vi "test-Coordinate-System-Test2.vi"() -> (3 "All tests passed":bool)   [LabVIEW 2019]
uses:
  <vilib>/Rock Robotics/WPI/ThirdParty/JAS_Junk/TrajLib/CoordAxis_N.vi
  <vilib>/Rock Robotics/WPI/ThirdParty/JAS_Junk/TrajLib/CoordSystem_New.vi
  <vilib>/Rock Robotics/WPI/ThirdParty/JAS_Junk/TrajLib/CoordAxis_E.vi
  <vilib>/Rock Robotics/WPI/ThirdParty/JAS_Junk/TrajLib/CoordAxis_D.vi
  <vilib>/Rock Robotics/WPI/ThirdParty/JAS_Junk/TrajLib/Conv_Deg_Radians.vi
  <vilib>/Rock Robotics/WPI/ThirdParty/JAS_Junk/TrajLib/Quaternion_New.vi
  <vilib>/Rock Robotics/WPI/ThirdParty/JAS_Junk/TrajLib/Translation3d_Create.vi
  <vilib>/Rock Robotics/WPI/ThirdParty/JAS_Junk/TrajLib/Pose3d_New_Trans3dRot3d.vi
  <vilib>/Rock Robotics/WPI/ThirdParty/JAS_Junk/TrajLib/Rotation3d_Minus.vi
  <vilib>/Rock Robotics/WPI/ThirdParty/JAS_Junk/TrajLib/Translation3d_Create_Default.vi
  <vilib>/Rock Robotics/WPI/ThirdParty/JAS_Junk/TrajLib/Pose3d_RelativeTo.vi
  <vilib>/Rock Robotics/WPI/ThirdParty/JAS_Junk/TrajLib/CoordAxis_New.vi
  <vilib>/Rock Robotics/WPI/ThirdParty/JAS_Junk/TrajLib/MatBuilder_Create.vi
  <vilib>/Rock Robotics/WPI/ThirdParty/JAS_Junk/TrajLib/Matrix_AssignBlock.vi
  <vilib>/Rock Robotics/WPI/ThirdParty/JAS_Junk/TrajLib/Matrix_Transpose.vi
  <vilib>/Rock Robotics/WPI/ThirdParty/JAS_Junk/TrajLib/Matrix_Ident.vi
  <vilib>/Rock Robotics/WPI/ThirdParty/JAS_Junk/TrajLib/Matrix_IsEqual.vi
  <vilib>/Analysis/baseanly.llb/A x B.vi
  <vilib>/Analysis/baseanly.llb/Real A x B.vi
  <vilib>/Rock Robotics/WPI/ThirdParty/JAS_Junk/TrajLib/Rotation3d_Create_Quaternion.vi
  <vilib>/Rock Robotics/WPI/ThirdParty/JAS_Junk/TrajLib/Rotation3d_UnaryMinus.vi
  <vilib>/Rock Robotics/WPI/ThirdParty/JAS_Junk/TrajLib/Rotation3d_RotateBy.vi
  <vilib>/Rock Robotics/WPI/ThirdParty/JAS_Junk/TrajLib/Transform3d_Create_Pose3dPose3d.vi
  <vilib>/Rock Robotics/WPI/ThirdParty/JAS_Junk/TrajLib/Transform3d_GetRotation3d.vi
  <vilib>/Rock Robotics/WPI/ThirdParty/JAS_Junk/TrajLib/Transform3d_GetTranslation3d.vi
  <vilib>/Rock Robotics/WPI/ThirdParty/JAS_Junk/TrajLib/Rotation3d_GetQuaterion.vi
  <vilib>/Rock Robotics/WPI/ThirdParty/JAS_Junk/TrajLib/Quaternion_Equals.vi
  <vilib>/Rock Robotics/WPI/ThirdParty/JAS_Junk/TrajLib/MatrixHelper_CoerceSize.vi
  <vilib>/Rock Robotics/WPI/ThirdParty/JAS_Junk/TrajLib/Quaternion_Normalize.vi
  <vilib>/Rock Robotics/WPI/ThirdParty/JAS_Junk/TrajLib/Quaternion_Inverse.vi
  <vilib>/Rock Robotics/WPI/ThirdParty/JAS_Junk/TrajLib/Quaternion_Times.vi
  <vilib>/Rock Robotics/WPI/ThirdParty/JAS_Junk/TrajLib/Transform3d_Create_Trans3dRot3d.vi
  <vilib>/Rock Robotics/WPI/ThirdParty/JAS_Junk/TrajLib/Translation3d_Minus.vi
  <vilib>/Rock Robotics/WPI/ThirdParty/JAS_Junk/TrajLib/Translation3d_RotateBy.vi
  <vilib>/Rock Robotics/WPI/ThirdParty/JAS_Junk/TrajLib/Quaternion_New_Default.vi
  <vilib>/Rock Robotics/WPI/ThirdParty/JAS_Junk/TrajLib/Quaternion_Get_All.vi
  <vilib>/Analysis/7linalg.llb/Create Special Matrix.vi
  <vilib>/Analysis/7linalg.llb/Create Special Real Matrix.vi
  <vilib>/Analysis/Matrix/Numeric/Conversions/Array To Matrix.vi
  <vilib>/Analysis/Matrix/Numeric/Conversions/Array To Matrix - RA.vi
  <vilib>/Rock Robotics/WPI/ThirdParty/JAS_Junk/TrajLib/Trajectory_Library.lvlib
panel:
  out "Test 4":bool
  out "Test 3":bool
  out "Test 2":bool
  out "Test 1":bool
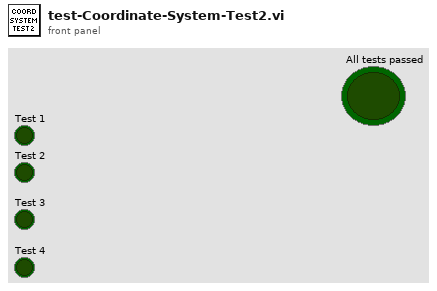
[diagram p1: front panel]
types:
  T1 = typedef "Trajectory_Library.lvlib/ROTATION3D.ctl" = cluster{"Q_quaternion":T2}
  T2 = typedef "Trajectory_Library.lvlib/QUATERNION.ctl" = cluster{"R":dbl, "V":dbl[]}
  T3 = typedef "Trajectory_Library.lvlib/POSE3D.ctl" = cluster{"Translation3d":T4, "Rotation3d":T1}
  T4 = typedef "Trajectory_Library.lvlib/TRANSLATION3D.ctl" = cluster{"X":dbl, "Y":dbl, "Z":dbl}
  T5 = typedef "Trajectory_Library.lvlib/COORDINATE_SYSTEM.ctl" = cluster{"Rotation":T1}
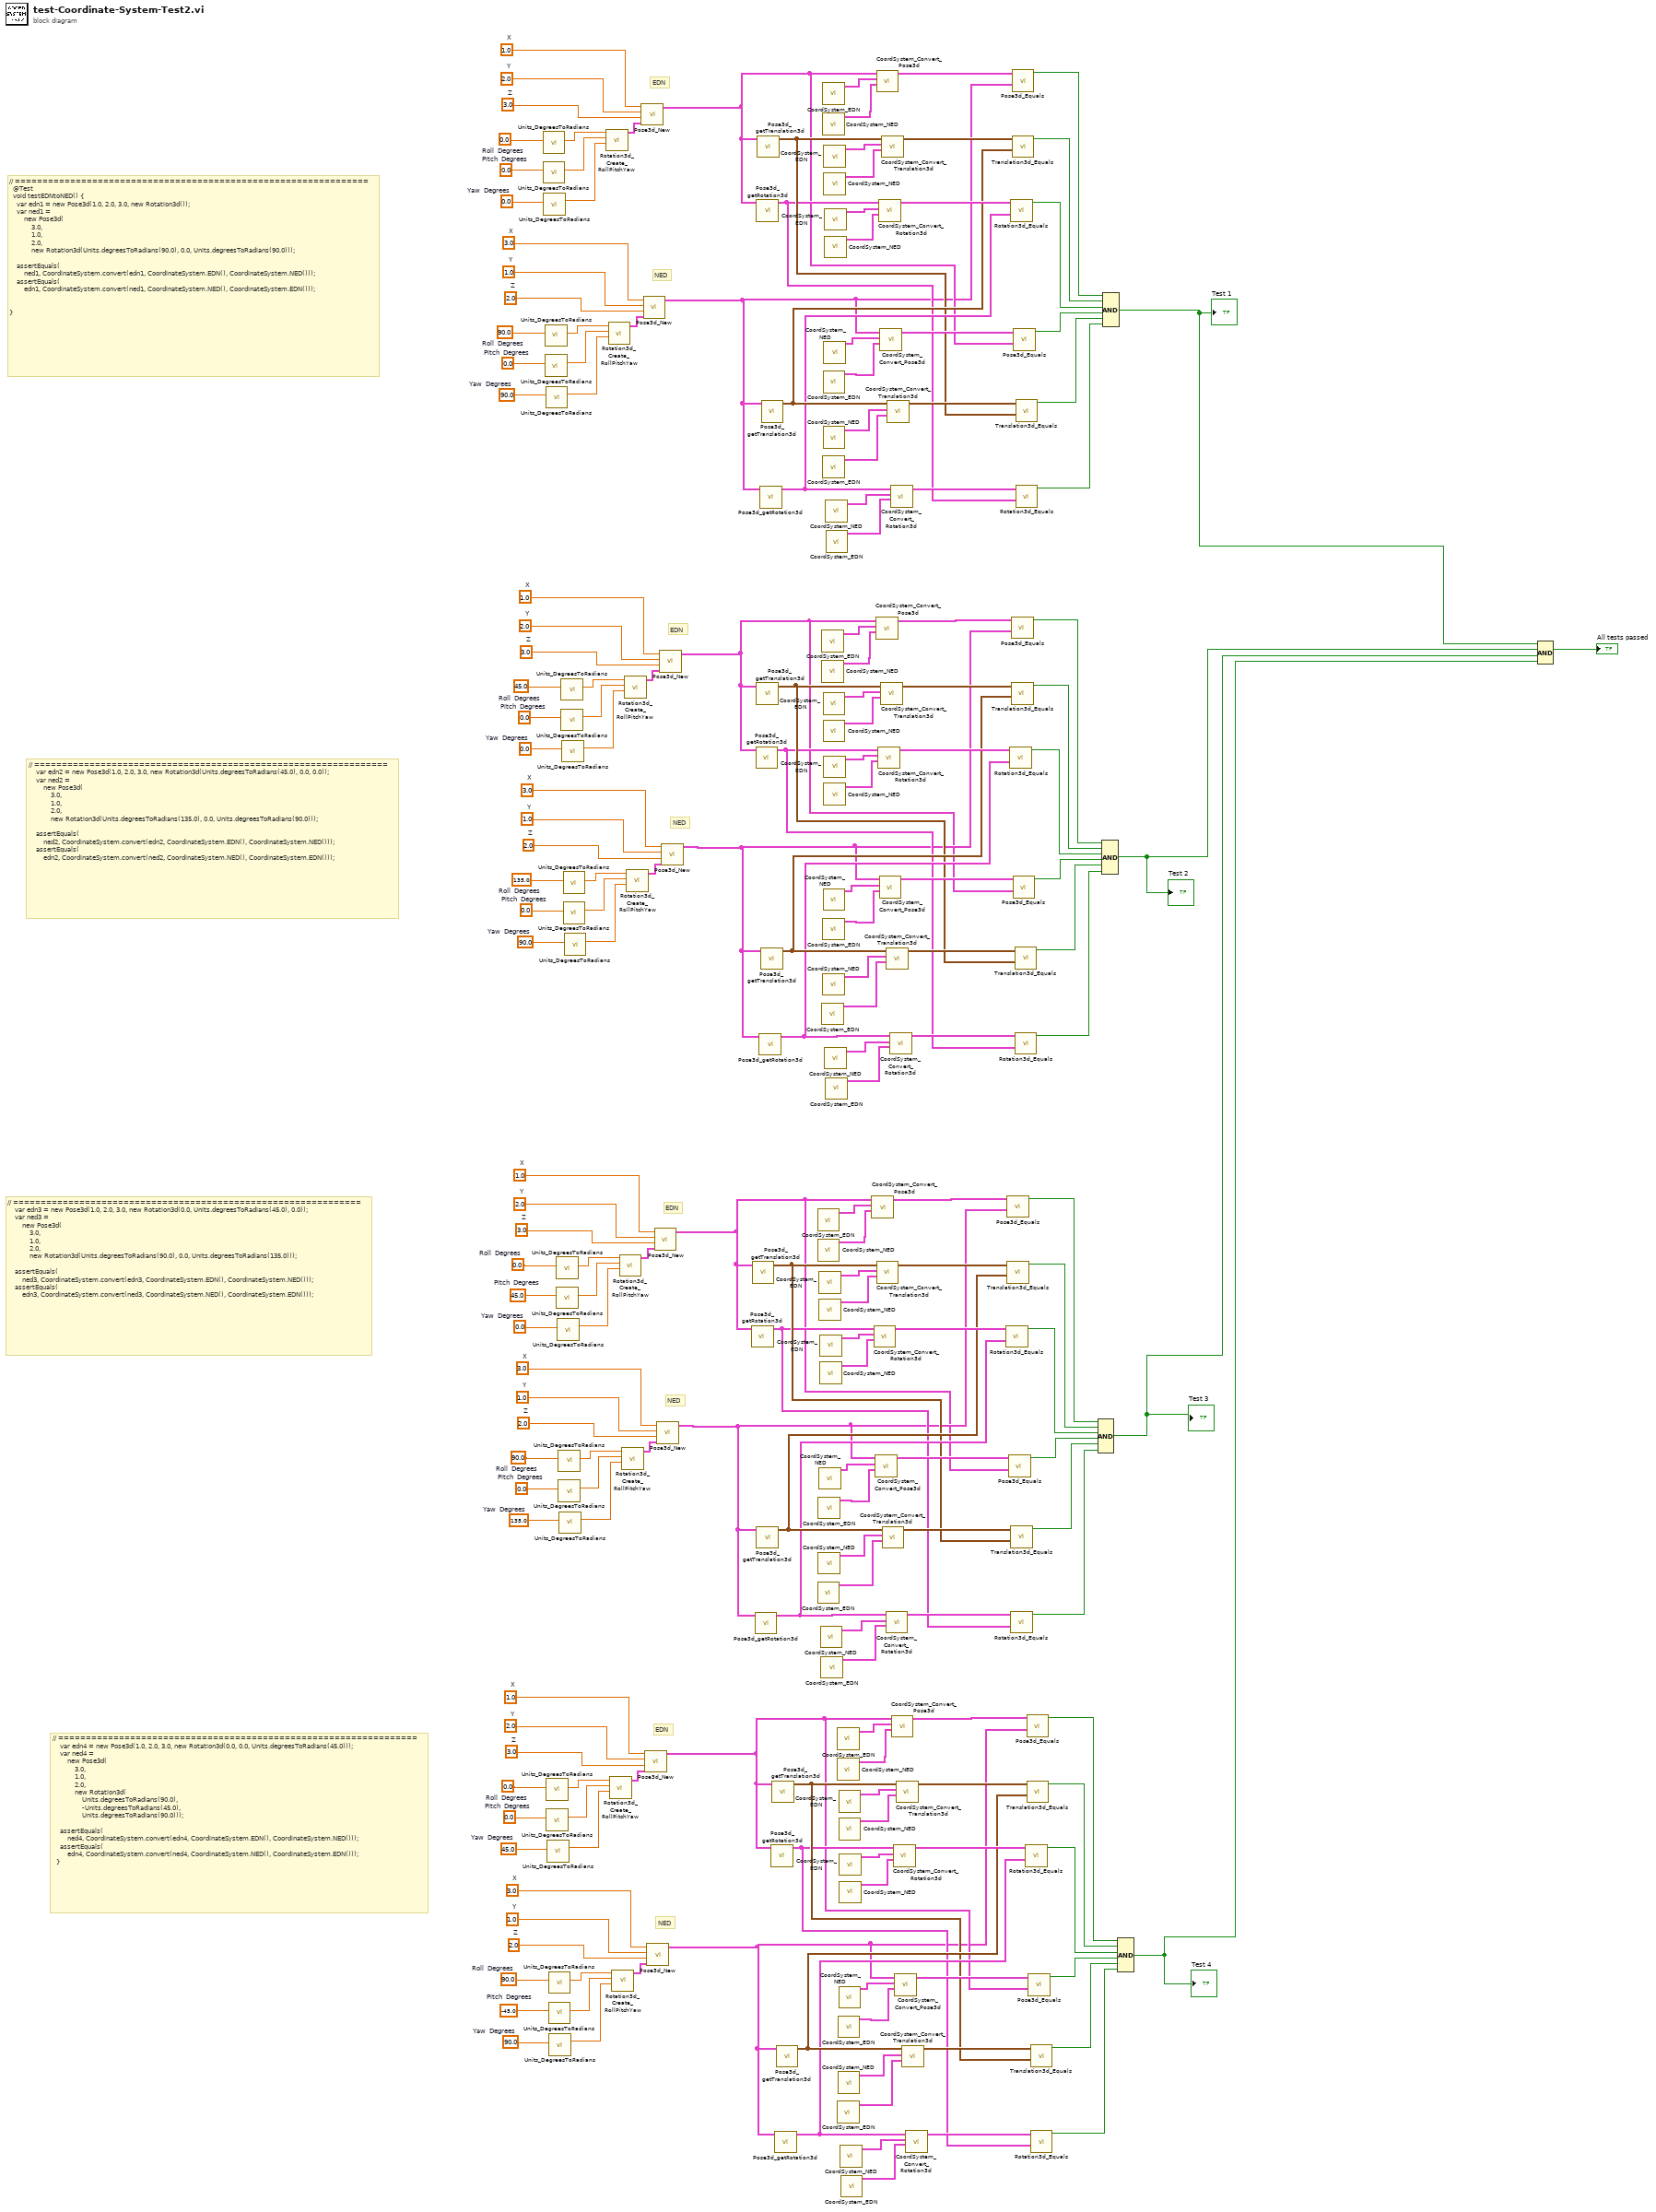
[diagram p0: block diagram]
diagram:
  w133 = 3.0  # X
  w132 = 1.0  # Y
  w131 = 2.0  # Z
  w125 = 90.0  # Roll  Degrees
  w126 = -45.0  # Pitch  Degrees
  w127 = 90.0  # Yaw  Degrees
  w143 = 1.0  # X
  w142 = 2.0  # Y
  w141 = 3.0  # Z
  w135 = 0.0  # Roll  Degrees
  w136 = 0.0  # Pitch  Degrees
  w137 = 45.0  # Yaw  Degrees
  w153 = 3.0  # X
  w152 = 1.0  # Y
  w151 = 2.0  # Z
  w145 = 90.0  # Roll  Degrees
  w146 = 0.0  # Pitch  Degrees
  w147 = 135.0  # Yaw  Degrees
  w163 = 1.0  # X
  w162 = 2.0  # Y
  w161 = 3.0  # Z
  w155 = 0.0  # Roll  Degrees
  w156 = 45.0  # Pitch  Degrees
  w157 = 0.0  # Yaw  Degrees
  w173 = 3.0  # X
  w172 = 1.0  # Y
  w171 = 2.0  # Z
  w165 = 135.0  # Roll  Degrees
  w166 = 0.0  # Pitch  Degrees
  w167 = 90.0  # Yaw  Degrees
  w183 = 1.0  # X
  w182 = 2.0  # Y
  w181 = 3.0  # Z
  w175 = 45.0  # Roll  Degrees
  w176 = 0.0  # Pitch  Degrees
  w177 = 0.0  # Yaw  Degrees
  w194 = 3.0  # X
  w193 = 1.0  # Y
  w192 = 2.0  # Z
  w186 = 90.0  # Roll  Degrees
  w187 = 0.0  # Pitch  Degrees
  w188 = 90.0  # Yaw  Degrees
  w204 = 1.0  # X
  w203 = 2.0  # Y
  w202 = 3.0  # Z
  w196 = 0.0  # Roll  Degrees
  w197 = 0.0  # Pitch  Degrees
  w198 = 0.0  # Yaw  Degrees
  # "NED"
  # "EDN"
  # "NED"
  # "EDN"
  # "// ================================================================\n    var edn2 = new Pose3d(1.0, 2.0, 3.0, new Rotation3d(Units.degreesToRadians(45.0), 0.0, 0.0));\n    var ned2 =\n        new Pose3d(\n            3.0,\n            1.0,\n            2.0,\n            new Rotation3d(Units.degreesToRadians(135.0), 0.0, Units.degreesToRadians(90.0)));\n\n    assertEquals(\n        ned2, CoordinateSystem.convert(edn2, CoordinateSystem.EDN(), CoordinateSystem.NED()));\n    assertEquals(\n        edn2, CoordinateSystem.convert(ned2, CoordinateSystem.NED(), CoordinateSystem.EDN()));"
  # "// ===============================================================\n    var edn3 = new Pose3d(1.0, 2.0, 3.0, new Rotation3d(0.0, Units.degreesToRadians(45.0), 0.0));\n    var ned3 =\n        new Pose3d(\n            3.0,\n            1.0,\n            2.0,\n            new Rotation3d(Units.degreesToRadians(90.0), 0.0, Units.degreesToRadians(135.0)));\n\n    assertEquals(\n        ned3, CoordinateSystem.convert(edn3, CoordinateSystem.EDN(), CoordinateSystem.NED()));\n    assertEquals(\n        edn3, CoordinateSystem.convert(ned3, CoordinateSystem.NED(), CoordinateSystem.EDN()));"
  # "// =================================================================\n    var edn4 = new Pose3d(1.0, 2.0, 3.0, new Rotation3d(0.0, 0.0, Units.degreesToRadians(45.0)));\n    var ned4 =\n        new Pose3d(\n            3.0,\n            1.0,\n            2.0,\n            new Rotation3d(\n                Units.degreesToRadians(90.0),\n                -Units.degreesToRadians(45.0),\n                Units.degreesToRadians(90.0)));\n\n    assertEquals(\n        ned4, CoordinateSystem.convert(edn4, CoordinateSystem.EDN(), CoordinateSystem.NED()));\n    assertEquals(\n        edn4, CoordinateSystem.convert(ned4, CoordinateSystem.NED(), CoordinateSystem.EDN()));\n  }"
  # "NED"
  # "EDN"
  # "// ================================================================\n  @Test\n  void testEDNtoNED() {\n    var edn1 = new Pose3d(1.0, 2.0, 3.0, new Rotation3d());\n    var ned1 =\n        new Pose3d(\n            3.0,\n            1.0,\n            2.0,\n            new Rotation3d(Units.degreesToRadians(90.0), 0.0, Units.degreesToRadians(90.0)));\n\n    assertEquals(\n        ned1, CoordinateSystem.convert(edn1, CoordinateSystem.EDN(), CoordinateSystem.NED()));\n    assertEquals(\n        edn1, CoordinateSystem.convert(ned1, CoordinateSystem.NED(), CoordinateSystem.EDN()));\n\n\n}"
  # "NED"
  # "EDN"
  n1 = call <vilib>:"Units_DegreesToRadians.vi"("Degrees"=w196) -> ("Radians"=w199:dbl)  [unwired: 10 in]
  n2 = call <vilib>:"Units_DegreesToRadians.vi"("Degrees"=w197) -> ("Radians"=w200:dbl)  [unwired: 10 in]
  n3 = call <vilib>:"Units_DegreesToRadians.vi"("Degrees"=w198) -> ("Radians"=w201:dbl)  [unwired: 10 in]
  n4 = call <vilib>:"Units_DegreesToRadians.vi"("Degrees"=w186) -> ("Radians"=w189:dbl)  [unwired: 10 in]
  n5 = call <vilib>:"Units_DegreesToRadians.vi"("Degrees"=w187) -> ("Radians"=w190:dbl)  [unwired: 10 in]
  n6 = call <vilib>:"Units_DegreesToRadians.vi"("Degrees"=w188) -> ("Radians"=w191:dbl)  [unwired: 10 in]
  n7 = call <vilib>:"Units_DegreesToRadians.vi"("Degrees"=w135) -> ("Radians"=w138:dbl)  [unwired: 10 in]
  n8 = call <vilib>:"Units_DegreesToRadians.vi"("Degrees"=w136) -> ("Radians"=w139:dbl)  [unwired: 10 in]
  n9 = call <vilib>:"Units_DegreesToRadians.vi"("Degrees"=w137) -> ("Radians"=w140:dbl)  [unwired: 10 in]
  n10 = call <vilib>:"Units_DegreesToRadians.vi"("Degrees"=w125) -> ("Radians"=w128:dbl)  [unwired: 10 in]
  n11 = call <vilib>:"Units_DegreesToRadians.vi"("Degrees"=w126) -> ("Radians"=w129:dbl)  [unwired: 10 in]
  n12 = call <vilib>:"Units_DegreesToRadians.vi"("Degrees"=w127) -> ("Radians"=w130:dbl)  [unwired: 10 in]
  n13 = call <vilib>:"Units_DegreesToRadians.vi"("Degrees"=w155) -> ("Radians"=w158:dbl)  [unwired: 10 in]
  n14 = call <vilib>:"Units_DegreesToRadians.vi"("Degrees"=w156) -> ("Radians"=w159:dbl)  [unwired: 10 in]
  n15 = call <vilib>:"Units_DegreesToRadians.vi"("Degrees"=w157) -> ("Radians"=w160:dbl)  [unwired: 10 in]
  n16 = call <vilib>:"Units_DegreesToRadians.vi"("Degrees"=w145) -> ("Radians"=w148:dbl)  [unwired: 10 in]
  n17 = call <vilib>:"Units_DegreesToRadians.vi"("Degrees"=w146) -> ("Radians"=w149:dbl)  [unwired: 10 in]
  n18 = call <vilib>:"Units_DegreesToRadians.vi"("Degrees"=w147) -> ("Radians"=w150:dbl)  [unwired: 10 in]
  n19 = call <vilib>:"Units_DegreesToRadians.vi"("Degrees"=w175) -> ("Radians"=w178:dbl)  [unwired: 10 in]
  n20 = call <vilib>:"Units_DegreesToRadians.vi"("Degrees"=w176) -> ("Radians"=w179:dbl)  [unwired: 10 in]
  n21 = call <vilib>:"Units_DegreesToRadians.vi"("Degrees"=w177) -> ("Radians"=w180:dbl)  [unwired: 10 in]
  n22 = call <vilib>:"Units_DegreesToRadians.vi"("Degrees"=w165) -> ("Radians"=w168:dbl)  [unwired: 10 in]
  n23 = call <vilib>:"Units_DegreesToRadians.vi"("Degrees"=w166) -> ("Radians"=w169:dbl)  [unwired: 10 in]
  n24 = call <vilib>:"Units_DegreesToRadians.vi"("Degrees"=w167) -> ("Radians"=w170:dbl)  [unwired: 10 in]
  n25 = call <vilib>:"Rotation3d_Create_RollPitchYaw.vi"("Yaw"=w201, "Pitch"=w200, "Roll"=w199) -> ("Rotation3d"=w205:T1)  [unwired: 8 in]
  n26 = call <vilib>:"Rotation3d_Create_RollPitchYaw.vi"("Yaw"=w191, "Pitch"=w190, "Roll"=w189) -> ("Rotation3d"=w195:T1)  [unwired: 8 in]
  n27 = call <vilib>:"Rotation3d_Create_RollPitchYaw.vi"("Yaw"=w140, "Pitch"=w139, "Roll"=w138) -> ("Rotation3d"=w144:T1)  [unwired: 8 in]
  n28 = call <vilib>:"Rotation3d_Create_RollPitchYaw.vi"("Yaw"=w130, "Pitch"=w129, "Roll"=w128) -> ("Rotation3d"=w134:T1)  [unwired: 8 in]
  n29 = call <vilib>:"Rotation3d_Create_RollPitchYaw.vi"("Yaw"=w160, "Pitch"=w159, "Roll"=w158) -> ("Rotation3d"=w164:T1)  [unwired: 8 in]
  n30 = call <vilib>:"Rotation3d_Create_RollPitchYaw.vi"("Yaw"=w150, "Pitch"=w149, "Roll"=w148) -> ("Rotation3d"=w154:T1)  [unwired: 8 in]
  n31 = call <vilib>:"Rotation3d_Create_RollPitchYaw.vi"("Yaw"=w180, "Pitch"=w179, "Roll"=w178) -> ("Rotation3d"=w184:T1)  [unwired: 8 in]
  n32 = call <vilib>:"Rotation3d_Create_RollPitchYaw.vi"("Yaw"=w170, "Pitch"=w169, "Roll"=w168) -> ("Rotation3d"=w174:T1)  [unwired: 8 in]
  n33 = call <vilib>:"Pose3d_New.vi"("Rotation3d"=w205, "z"=w202, "Y"=w203, "X"=w204) -> ("out Pose3d"=w3:T3)  [unwired: 7 in]
  n34 = call <vilib>:"Pose3d_New.vi"("Rotation3d"=w195, "z"=w192, "Y"=w193, "X"=w194) -> ("out Pose3d"=w2:T3)  [unwired: 7 in]
  n35 = call <vilib>:"Pose3d_New.vi"("Rotation3d"=w144, "z"=w141, "Y"=w142, "X"=w143) -> ("out Pose3d"=w96:T3)  [unwired: 7 in]
  n36 = call <vilib>:"Pose3d_New.vi"("Rotation3d"=w134, "z"=w131, "Y"=w132, "X"=w133) -> ("out Pose3d"=w95:T3)  [unwired: 7 in]
  n37 = call <vilib>:"Pose3d_New.vi"("Rotation3d"=w164, "z"=w161, "Y"=w162, "X"=w163) -> ("out Pose3d"=w64:T3)  [unwired: 7 in]
  n38 = call <vilib>:"Pose3d_New.vi"("Rotation3d"=w154, "z"=w151, "Y"=w152, "X"=w153) -> ("out Pose3d"=w65:T3)  [unwired: 7 in]
  n39 = call <vilib>:"Pose3d_New.vi"("Rotation3d"=w184, "z"=w181, "Y"=w182, "X"=w183) -> ("out Pose3d"=w33:T3)  [unwired: 7 in]
  n40 = call <vilib>:"Pose3d_New.vi"("Rotation3d"=w174, "z"=w171, "Y"=w172, "X"=w173) -> ("out Pose3d"=w34:T3)  [unwired: 7 in]
  n41 = call <vilib>:"Pose3d_getRotation3d.vi"("in Pose3d"=w64) -> ("out Rotation3d"=w83:T1)  [unwired: 10 in]
  n42 = call <vilib>:"Pose3d_getTranslation3d.vi"("in Pose3d"=w64) -> ("out Translation3d"=w84:T4)  [unwired: 10 in]
  n43 = call <vilib>:"Pose3d_getRotation3d.vi"("in Pose3d"=w65) -> ("out Rotation3d"=w85:T1)  [unwired: 10 in]
  n44 = call <vilib>:"Pose3d_getRotation3d.vi"("in Pose3d"=w33) -> ("out Rotation3d"=w52:T1)  [unwired: 10 in]
  n45 = call <vilib>:"Pose3d_getRotation3d.vi"("in Pose3d"=w3) -> ("out Rotation3d"=w21:T1)  [unwired: 10 in]
  n46 = call <vilib>:"Pose3d_getTranslation3d.vi"("in Pose3d"=w33) -> ("out Translation3d"=w53:T4)  [unwired: 10 in]
  n47 = call <vilib>:"Pose3d_getTranslation3d.vi"("in Pose3d"=w65) -> ("out Translation3d"=w86:T4)  [unwired: 10 in]
  n48 = call <vilib>:"Pose3d_getTranslation3d.vi"("in Pose3d"=w3) -> ("out Translation3d"=w22:T4)  [unwired: 10 in]
  n49 = call <vilib>:"Pose3d_getRotation3d.vi"("in Pose3d"=w34) -> ("out Rotation3d"=w54:T1)  [unwired: 10 in]
  n50 = call <vilib>:"Pose3d_getRotation3d.vi"("in Pose3d"=w2) -> ("out Rotation3d"=w23:T1)  [unwired: 10 in]
  n51 = call <vilib>:"Pose3d_getTranslation3d.vi"("in Pose3d"=w34) -> ("out Translation3d"=w55:T4)  [unwired: 10 in]
  n52 = call <vilib>:"Pose3d_getTranslation3d.vi"("in Pose3d"=w2) -> ("out Translation3d"=w24:T4)  [unwired: 10 in]
  n53 = call <vilib>:"Pose3d_getRotation3d.vi"("in Pose3d"=w96) -> ("out Rotation3d"=w114:T1)  [unwired: 10 in]
  n54 = call <vilib>:"Pose3d_getTranslation3d.vi"("in Pose3d"=w96) -> ("out Translation3d"=w115:T4)  [unwired: 10 in]
  n55 = call <vilib>:"Pose3d_getRotation3d.vi"("in Pose3d"=w95) -> ("out Rotation3d"=w116:T1)  [unwired: 10 in]
  n56 = call <vilib>:"Pose3d_getTranslation3d.vi"("in Pose3d"=w95) -> ("out Translation3d"=w117:T4)  [unwired: 10 in]
  n57 = call <vilib>:"CoordSystem_EDN.vi"() -> ("out Coordinate System"=w77:T5)  [unwired: 10 in, 1 out]
  n58 = call <vilib>:"CoordSystem_NED.vi"() -> ("out Coordinate System"=w76:T5)  [unwired: 10 in, 1 out]
  n59 = call <vilib>:"CoordSystem_EDN.vi"() -> ("out Coordinate System"=w68:T5)  [unwired: 10 in, 1 out]
  n60 = call <vilib>:"CoordSystem_EDN.vi"() -> ("out Coordinate System"=w70:T5)  [unwired: 10 in, 1 out]
  n61 = call <vilib>:"CoordSystem_NED.vi"() -> ("out Coordinate System"=w69:T5)  [unwired: 10 in, 1 out]
  n62 = call <vilib>:"CoordSystem_EDN.vi"() -> ("out Coordinate System"=w75:T5)  [unwired: 10 in, 1 out]
  n63 = call <vilib>:"CoordSystem_NED.vi"() -> ("out Coordinate System"=w74:T5)  [unwired: 10 in, 1 out]
  n64 = call <vilib>:"CoordSystem_NED.vi"() -> ("out Coordinate System"=w71:T5)  [unwired: 10 in, 1 out]
  n65 = call <vilib>:"CoordSystem_EDN.vi"() -> ("out Coordinate System"=w73:T5)  [unwired: 10 in, 1 out]
  n66 = call <vilib>:"CoordSystem_NED.vi"() -> ("out Coordinate System"=w72:T5)  [unwired: 10 in, 1 out]
  n67 = call <vilib>:"CoordSystem_NED.vi"() -> ("out Coordinate System"=w67:T5)  [unwired: 10 in, 1 out]
  n68 = call <vilib>:"CoordSystem_EDN.vi"() -> ("out Coordinate System"=w66:T5)  [unwired: 10 in, 1 out]
  n69 = call <vilib>:"CoordSystem_EDN.vi"() -> ("out Coordinate System"=w46:T5)  [unwired: 10 in, 1 out]
  n70 = call <vilib>:"CoordSystem_NED.vi"() -> ("out Coordinate System"=w45:T5)  [unwired: 10 in, 1 out]
  n71 = call <vilib>:"CoordSystem_EDN.vi"() -> ("out Coordinate System"=w37:T5)  [unwired: 10 in, 1 out]
  n72 = call <vilib>:"CoordSystem_EDN.vi"() -> ("out Coordinate System"=w15:T5)  [unwired: 10 in, 1 out]
  n73 = call <vilib>:"CoordSystem_NED.vi"() -> ("out Coordinate System"=w14:T5)  [unwired: 10 in, 1 out]
  n74 = call <vilib>:"CoordSystem_EDN.vi"() -> ("out Coordinate System"=w6:T5)  [unwired: 10 in, 1 out]
  n75 = call <vilib>:"CoordSystem_EDN.vi"() -> ("out Coordinate System"=w39:T5)  [unwired: 10 in, 1 out]
  n76 = call <vilib>:"CoordSystem_NED.vi"() -> ("out Coordinate System"=w38:T5)  [unwired: 10 in, 1 out]
  n77 = call <vilib>:"CoordSystem_EDN.vi"() -> ("out Coordinate System"=w8:T5)  [unwired: 10 in, 1 out]
  n78 = call <vilib>:"CoordSystem_NED.vi"() -> ("out Coordinate System"=w7:T5)  [unwired: 10 in, 1 out]
  n79 = call <vilib>:"CoordSystem_EDN.vi"() -> ("out Coordinate System"=w44:T5)  [unwired: 10 in, 1 out]
  n80 = call <vilib>:"CoordSystem_NED.vi"() -> ("out Coordinate System"=w43:T5)  [unwired: 10 in, 1 out]
  n81 = call <vilib>:"CoordSystem_NED.vi"() -> ("out Coordinate System"=w40:T5)  [unwired: 10 in, 1 out]
  n82 = call <vilib>:"CoordSystem_EDN.vi"() -> ("out Coordinate System"=w13:T5)  [unwired: 10 in, 1 out]
  n83 = call <vilib>:"CoordSystem_NED.vi"() -> ("out Coordinate System"=w12:T5)  [unwired: 10 in, 1 out]
  n84 = call <vilib>:"CoordSystem_NED.vi"() -> ("out Coordinate System"=w9:T5)  [unwired: 10 in, 1 out]
  n85 = call <vilib>:"CoordSystem_EDN.vi"() -> ("out Coordinate System"=w42:T5)  [unwired: 10 in, 1 out]
  n86 = call <vilib>:"CoordSystem_NED.vi"() -> ("out Coordinate System"=w41:T5)  [unwired: 10 in, 1 out]
  n87 = call <vilib>:"CoordSystem_EDN.vi"() -> ("out Coordinate System"=w11:T5)  [unwired: 10 in, 1 out]
  n88 = call <vilib>:"CoordSystem_NED.vi"() -> ("out Coordinate System"=w10:T5)  [unwired: 10 in, 1 out]
  n89 = call <vilib>:"CoordSystem_NED.vi"() -> ("out Coordinate System"=w36:T5)  [unwired: 10 in, 1 out]
  n90 = call <vilib>:"CoordSystem_NED.vi"() -> ("out Coordinate System"=w5:T5)  [unwired: 10 in, 1 out]
  n91 = call <vilib>:"CoordSystem_EDN.vi"() -> ("out Coordinate System"=w35:T5)  [unwired: 10 in, 1 out]
  n92 = call <vilib>:"CoordSystem_EDN.vi"() -> ("out Coordinate System"=w4:T5)  [unwired: 10 in, 1 out]
  n93 = call <vilib>:"CoordSystem_EDN.vi"() -> ("out Coordinate System"=w108:T5)  [unwired: 10 in, 1 out]
  n94 = call <vilib>:"CoordSystem_NED.vi"() -> ("out Coordinate System"=w107:T5)  [unwired: 10 in, 1 out]
  n95 = call <vilib>:"CoordSystem_EDN.vi"() -> ("out Coordinate System"=w99:T5)  [unwired: 10 in, 1 out]
  n96 = call <vilib>:"CoordSystem_EDN.vi"() -> ("out Coordinate System"=w101:T5)  [unwired: 10 in, 1 out]
  n97 = call <vilib>:"CoordSystem_NED.vi"() -> ("out Coordinate System"=w100:T5)  [unwired: 10 in, 1 out]
  n98 = call <vilib>:"CoordSystem_EDN.vi"() -> ("out Coordinate System"=w106:T5)  [unwired: 10 in, 1 out]
  n99 = call <vilib>:"CoordSystem_NED.vi"() -> ("out Coordinate System"=w105:T5)  [unwired: 10 in, 1 out]
  n100 = call <vilib>:"CoordSystem_NED.vi"() -> ("out Coordinate System"=w102:T5)  [unwired: 10 in, 1 out]
  n101 = call <vilib>:"CoordSystem_EDN.vi"() -> ("out Coordinate System"=w104:T5)  [unwired: 10 in, 1 out]
  n102 = call <vilib>:"CoordSystem_NED.vi"() -> ("out Coordinate System"=w103:T5)  [unwired: 10 in, 1 out]
  n103 = call <vilib>:"CoordSystem_NED.vi"() -> ("out Coordinate System"=w98:T5)  [unwired: 10 in, 1 out]
  n104 = call <vilib>:"CoordSystem_EDN.vi"() -> ("out Coordinate System"=w97:T5)  [unwired: 10 in, 1 out]
  n105 = call <vilib>:"CoordSystem_Convert_Pose3d.vi"("CoordSys To"=w76, "CoordSys From"=w77, "in Pose3d"=w64) -> ("out Converted Pose3d"=w93:T3)  [unwired: 8 in]
  n106 = call <vilib>:"CoordSystem_Convert_Rotation3d.vi"("CoordSys To"=w72, "CoordSys From"=w73, "in Rotation3d"=w83) -> ("out Converted Rotation3d"=w89:T1)  [unwired: 8 in]
  n107 = call <vilib>:"CoordSystem_Convert_Pose3d.vi"("CoordSys To"=w70, "CoordSys From"=w71, "in Pose3d"=w65) -> ("out Converted Pose3d"=w92:T3)  [unwired: 8 in]
  n108 = call <vilib>:"CoordSystem_Convert_Pose3d.vi"("CoordSys To"=w45, "CoordSys From"=w46, "in Pose3d"=w33) -> ("out Converted Pose3d"=w62:T3)  [unwired: 8 in]
  n109 = call <vilib>:"CoordSystem_Convert_Pose3d.vi"("CoordSys To"=w14, "CoordSys From"=w15, "in Pose3d"=w3) -> ("out Converted Pose3d"=w31:T3)  [unwired: 8 in]
  n110 = call <vilib>:"CoordSystem_Convert_Translation3d.vi"("CoordSys To"=w74, "CoordSys From"=w75, "in Translation3d"=w84) -> ("out Converted Translation3d"=w90:T4)  [unwired: 8 in]
  n111 = call <vilib>:"CoordSystem_Convert_Rotation3d.vi"("CoordSys To"=w41, "CoordSys From"=w42, "in Rotation3d"=w52) -> ("out Converted Rotation3d"=w58:T1)  [unwired: 8 in]
  n112 = call <vilib>:"CoordSystem_Convert_Rotation3d.vi"("CoordSys To"=w10, "CoordSys From"=w11, "in Rotation3d"=w21) -> ("out Converted Rotation3d"=w27:T1)  [unwired: 8 in]
  n113 = call <vilib>:"CoordSystem_Convert_Pose3d.vi"("CoordSys To"=w39, "CoordSys From"=w40, "in Pose3d"=w34) -> ("out Converted Pose3d"=w61:T3)  [unwired: 8 in]
  n114 = call <vilib>:"CoordSystem_Convert_Pose3d.vi"("CoordSys To"=w8, "CoordSys From"=w9, "in Pose3d"=w2) -> ("out Converted Pose3d"=w30:T3)  [unwired: 8 in]
  n115 = call <vilib>:"CoordSystem_Convert_Translation3d.vi"("CoordSys To"=w43, "CoordSys From"=w44, "in Translation3d"=w53) -> ("out Converted Translation3d"=w59:T4)  [unwired: 8 in]
  n116 = call <vilib>:"CoordSystem_Convert_Translation3d.vi"("CoordSys To"=w12, "CoordSys From"=w13, "in Translation3d"=w22) -> ("out Converted Translation3d"=w28:T4)  [unwired: 8 in]
  n117 = call <vilib>:"CoordSystem_Convert_Translation3d.vi"("CoordSys To"=w68, "CoordSys From"=w69, "in Translation3d"=w86) -> ("out Converted Translation3d"=w88:T4)  [unwired: 8 in]
  n118 = call <vilib>:"CoordSystem_Convert_Rotation3d.vi"("CoordSys To"=w66, "CoordSys From"=w67, "in Rotation3d"=w85) -> ("out Converted Rotation3d"=w87:T1)  [unwired: 8 in]
  n119 = call <vilib>:"CoordSystem_Convert_Translation3d.vi"("CoordSys To"=w37, "CoordSys From"=w38, "in Translation3d"=w55) -> ("out Converted Translation3d"=w57:T4)  [unwired: 8 in]
  n120 = call <vilib>:"CoordSystem_Convert_Translation3d.vi"("CoordSys To"=w6, "CoordSys From"=w7, "in Translation3d"=w24) -> ("out Converted Translation3d"=w26:T4)  [unwired: 8 in]
  n121 = call <vilib>:"CoordSystem_Convert_Rotation3d.vi"("CoordSys To"=w35, "CoordSys From"=w36, "in Rotation3d"=w54) -> ("out Converted Rotation3d"=w56:T1)  [unwired: 8 in]
  n122 = call <vilib>:"CoordSystem_Convert_Rotation3d.vi"("CoordSys To"=w4, "CoordSys From"=w5, "in Rotation3d"=w23) -> ("out Converted Rotation3d"=w25:T1)  [unwired: 8 in]
  n123 = call <vilib>:"CoordSystem_Convert_Pose3d.vi"("CoordSys To"=w107, "CoordSys From"=w108, "in Pose3d"=w96) -> ("out Converted Pose3d"=w124:T3)  [unwired: 8 in]
  n124 = call <vilib>:"CoordSystem_Convert_Rotation3d.vi"("CoordSys To"=w103, "CoordSys From"=w104, "in Rotation3d"=w114) -> ("out Converted Rotation3d"=w120:T1)  [unwired: 8 in]
  n125 = call <vilib>:"CoordSystem_Convert_Pose3d.vi"("CoordSys To"=w101, "CoordSys From"=w102, "in Pose3d"=w95) -> ("out Converted Pose3d"=w123:T3)  [unwired: 8 in]
  n126 = call <vilib>:"CoordSystem_Convert_Translation3d.vi"("CoordSys To"=w105, "CoordSys From"=w106, "in Translation3d"=w115) -> ("out Converted Translation3d"=w121:T4)  [unwired: 8 in]
  n127 = call <vilib>:"CoordSystem_Convert_Translation3d.vi"("CoordSys To"=w99, "CoordSys From"=w100, "in Translation3d"=w117) -> ("out Converted Translation3d"=w119:T4)  [unwired: 8 in]
  n128 = call <vilib>:"CoordSystem_Convert_Rotation3d.vi"("CoordSys To"=w97, "CoordSys From"=w98, "in Rotation3d"=w116) -> ("out Converted Rotation3d"=w118:T1)  [unwired: 8 in]
  n129 = call <vilib>:"Rotation3d_Equals.vi"("other Rotation3d"=w85, "in Rotation3d"=w89) -> ("Equals"=w78:bool)  [unwired: 9 in]
  n130 = call <vilib>:"Pose3d_Equals.vi"("other Pose3d"=w65, "in Pose3d"=w93) -> ("Equals"=w80:bool)  [unwired: 9 in]
  n131 = call <vilib>:"Translation3d_Equals.vi"("other Translation3d"=w86, "In Translation3d"=w90) -> ("Equals"=w79:bool)  [unwired: 9 in]
  n132 = call <vilib>:"Pose3d_Equals.vi"("other Pose3d"=w64, "in Pose3d"=w92) -> ("Equals"=w91:bool)  [unwired: 9 in]
  n133 = call <vilib>:"Rotation3d_Equals.vi"("other Rotation3d"=w54, "in Rotation3d"=w58) -> ("Equals"=w47:bool)  [unwired: 9 in]
  n134 = call <vilib>:"Rotation3d_Equals.vi"("other Rotation3d"=w23, "in Rotation3d"=w27) -> ("Equals"=w16:bool)  [unwired: 9 in]
  n135 = call <vilib>:"Translation3d_Equals.vi"("other Translation3d"=w84, "In Translation3d"=w88) -> ("Equals"=w82:bool)  [unwired: 9 in]
  n136 = call <vilib>:"Rotation3d_Equals.vi"("other Rotation3d"=w83, "in Rotation3d"=w87) -> ("Equals"=w81:bool)  [unwired: 9 in]
  n137 = call <vilib>:"Pose3d_Equals.vi"("other Pose3d"=w34, "in Pose3d"=w62) -> ("Equals"=w49:bool)  [unwired: 9 in]
  n138 = call <vilib>:"Translation3d_Equals.vi"("other Translation3d"=w55, "In Translation3d"=w59) -> ("Equals"=w48:bool)  [unwired: 9 in]
  n139 = call <vilib>:"Pose3d_Equals.vi"("other Pose3d"=w2, "in Pose3d"=w31) -> ("Equals"=w18:bool)  [unwired: 9 in]
  n140 = call <vilib>:"Translation3d_Equals.vi"("other Translation3d"=w24, "In Translation3d"=w28) -> ("Equals"=w17:bool)  [unwired: 9 in]
  n141 = call <vilib>:"Pose3d_Equals.vi"("other Pose3d"=w33, "in Pose3d"=w61) -> ("Equals"=w60:bool)  [unwired: 9 in]
  n142 = call <vilib>:"Pose3d_Equals.vi"("other Pose3d"=w3, "in Pose3d"=w30) -> ("Equals"=w29:bool)  [unwired: 9 in]
  n143 = call <vilib>:"Translation3d_Equals.vi"("other Translation3d"=w53, "In Translation3d"=w57) -> ("Equals"=w51:bool)  [unwired: 9 in]
  n144 = call <vilib>:"Rotation3d_Equals.vi"("other Rotation3d"=w52, "in Rotation3d"=w56) -> ("Equals"=w50:bool)  [unwired: 9 in]
  n145 = call <vilib>:"Translation3d_Equals.vi"("other Translation3d"=w22, "In Translation3d"=w26) -> ("Equals"=w20:bool)  [unwired: 9 in]
  n146 = call <vilib>:"Rotation3d_Equals.vi"("other Rotation3d"=w21, "in Rotation3d"=w25) -> ("Equals"=w19:bool)  [unwired: 9 in]
  n147 = call <vilib>:"Rotation3d_Equals.vi"("other Rotation3d"=w116, "in Rotation3d"=w120) -> ("Equals"=w109:bool)  [unwired: 9 in]
  n148 = call <vilib>:"Pose3d_Equals.vi"("other Pose3d"=w95, "in Pose3d"=w124) -> ("Equals"=w111:bool)  [unwired: 9 in]
  n149 = call <vilib>:"Translation3d_Equals.vi"("other Translation3d"=w117, "In Translation3d"=w121) -> ("Equals"=w110:bool)  [unwired: 9 in]
  n150 = call <vilib>:"Pose3d_Equals.vi"("other Pose3d"=w96, "in Pose3d"=w123) -> ("Equals"=w122:bool)  [unwired: 9 in]
  n151 = call <vilib>:"Translation3d_Equals.vi"("other Translation3d"=w115, "In Translation3d"=w119) -> ("Equals"=w113:bool)  [unwired: 9 in]
  n152 = call <vilib>:"Rotation3d_Equals.vi"("other Rotation3d"=w114, "in Rotation3d"=w118) -> ("Equals"=w112:bool)  [unwired: 9 in]
  n153 = Compound Arithmetic op=AND(w80, w79, w78, w91, w82, w81) -> (w63:bool)
  "Test 3" <- w63
  n154 = Compound Arithmetic op=AND(w49, w48, w47, w60, w51, w50) -> (w32:bool)
  "Test 2" <- w32
  n155 = Compound Arithmetic op=AND(w18, w17, w16, w29, w20, w19) -> (w1:bool)
  "Test 1" <- w1
  n156 = Compound Arithmetic op=AND(w111, w110, w109, w122, w113, w112) -> (w94:bool)
  "Test 4" <- w94
  n157 = Compound Arithmetic op=AND(w1, w32, w63, w94) -> (→"All tests passed":bool)
